vi "Filter Library Owned Items.vi"(8 "Error In":errorcluster, 10 "Children[]":refnum<vi>[](array[refnum]), 11 "Library Project Item In":refnum<vi>) -> (0 "Error Out":errorcluster, 1 "Private Owned Items":refnum<vi>[](array[refnum]), 2 "Non-Private Owned Items":refnum<vi>[](array[refnum]), 3 "Library Project Item Out":refnum<vi>)   [LabVIEW 2018, in "Scripts.lvlib"]
uses:
  Scripts.lvlib
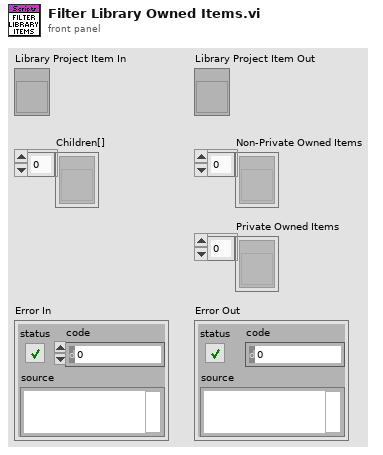
[diagram p1: front panel]
types:
  T1 = enum32{"invalid scope", "public", "private", "protected", "community"}
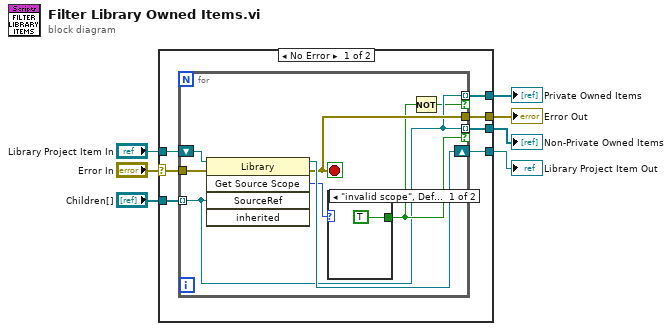
[diagram p0: block diagram]
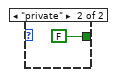
[diagram p2: hidden frame]
diagram:
  n1 = case shown="No Error" "Error In" {
    selector: "Error In" -> [w9 w25]
    tunnel: [w14 _] -> w7
    tunnel: [w13 _] -> w6
    tunnel: [w12 w25] -> w5
    tunnel: "Library Project Item In" -> [w8 w26]
    tunnel: [w11 w26] -> w2
    tunnel: "Children[]" -> [w10 _]
    frame No Error {
      n2 = for {
        shift-right: [w21] -> w11
        shift-left: w8 -> [w22]
        tunnel: w10 -> [w16] mode=indexing
        tunnel: w9 -> [w20]
        tunnel: [w19] -> w12
        tunnel: [w16] -> w14 mode=indexing if=w17
        tunnel: [w16] -> w13 mode=indexing if=w15
        stop <- w19 stop-if-true
        n3 = invoke class="Library" method="Get Source Scope"(reference=w22, error in=w20, "SourceRef"=w16) -> (reference out=w21:refnum<vi>, error out=w19:errorcluster, "GetSourceScope"=w18:T1)  [unwired: 2 in, 2 out]
        n4 = case shown="\"invalid scope\", Default" w18 {
          tunnel: [TRUE FALSE] -> w17
          frame "invalid scope", Default {
          }
          frame "private" {
          }
        }
        n5 = Not(x=w17) -> (.not. x?=w15:bool)
      }
    }
    frame Error {
    }
  }
  "Non-Private Owned Items" <- w7
  "Private Owned Items" <- w6
  "Error Out" <- w5
  "Library Project Item Out" <- w2
